vi "Linear Convert.vi"(6 "Inverse?":bool, 8 "Intercept":dbl, 9 "Slope":dbl, 11 "Signal":dbl) -> (3 "Result":dbl)   [LabVIEW 2016]
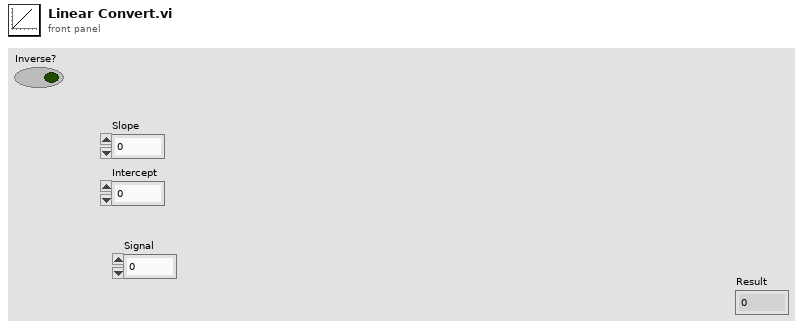
[diagram p1: front panel]
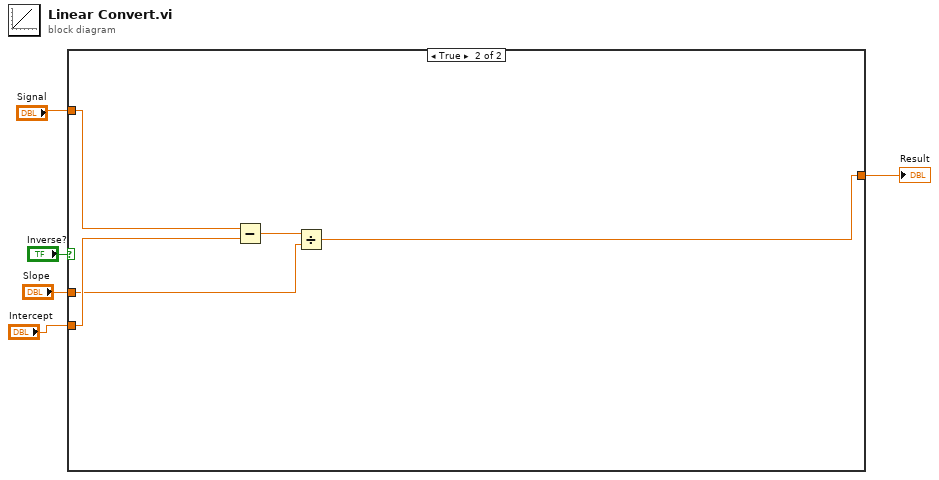
[diagram p0: block diagram]
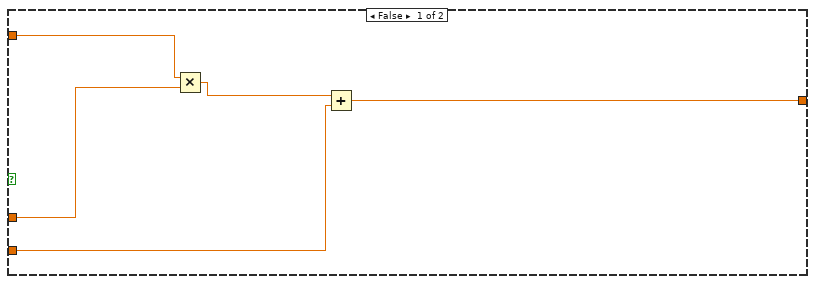
[diagram p2: hidden frame]
diagram:
  n1 = case shown="True" "Inverse?" {
    tunnel: [w9 w11] -> w4
    tunnel: "Signal" -> [w8 w15]
    tunnel: "Slope" -> [w7 w12]
    tunnel: "Intercept" -> [w6 w14]
    frame False {
      n2 = Multiply(x=w8, y=w7) -> (x*y=w10:dbl)
      n3 = Add(x=w10, y=w6) -> (x+y=w9:dbl)
    }
    frame True {
      n4 = Subtract(x=w15, y=w14) -> (x-y=w13:dbl)
      n5 = Divide(x=w13, y=w12) -> (x/y=w11:dbl)
    }
  }
  "Result" <- w4
